vi "Script Error.vi"(0 "Error?":bool, 1 "Reset Log":bool, 2 "Error Details":string, 3 "Error Code":i32, 4 "Line Number":i32) -> ()   [LabVIEW 2013]
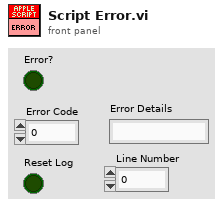
[diagram p1: front panel]
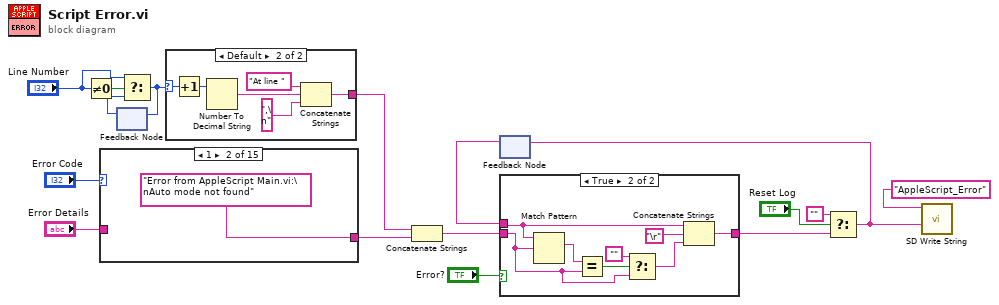
[diagram p0: block diagram]
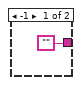
[diagram p2: hidden frame]
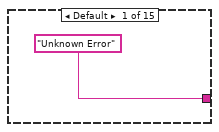
[diagram p4: hidden frame]
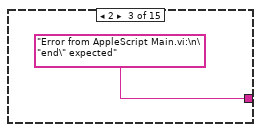
[diagram p5: hidden frame]
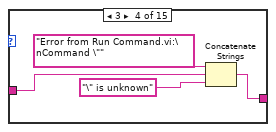
[diagram p6: hidden frame]
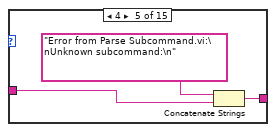
[diagram p7: hidden frame]
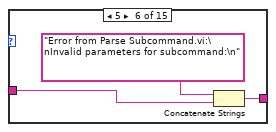
[diagram p8: hidden frame]
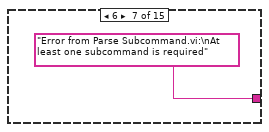
[diagram p9: hidden frame]
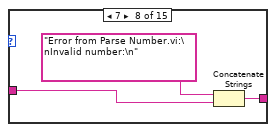
[diagram p10: hidden frame]
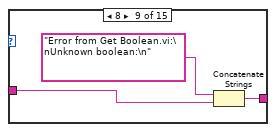
[diagram p11: hidden frame]
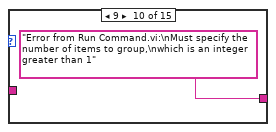
[diagram p12: hidden frame]
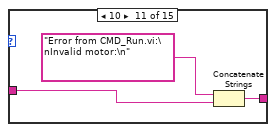
[diagram p13: hidden frame]
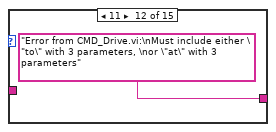
[diagram p14: hidden frame]
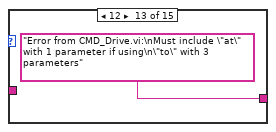
[diagram p15: hidden frame]
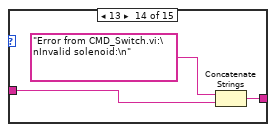
[diagram p16: hidden frame]
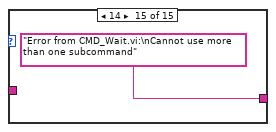
[diagram p17: hidden frame]
diagram:
  n1 = Not Equal To 0?(x="Line Number") -> (x != 0?=w4:bool)
  n2 = case shown="1" "Error Code" {
    tunnel: ["Unknown Error" "Error from AppleScript Main.vi:\nAuto mode not found" "Error from AppleScript Main.vi:\n\"end\" expected" w21 w24 w27 "Error from Parse Subcommand.vi:\nAt least one subcommand is required" w31 w34 "Error from Run Command.vi:\nMust specify the number of items to group,\nwhich is an integer greater than 1" w38 "Error from CMD_Drive.vi:\nMust include either \"to\" with 3 parameters, \nor \"at\" with 3 parameters" "Error from CMD_Drive.vi:\nMust include \"at\" with 1 parameter if using\n\"to\" with 3 parameters" w43 "Error from CMD_Wait.vi:\nCannot use more than one subcommand"] -> w9
    tunnel: "Error Details" -> [_ _ _ w22 w25 w28 _ w32 w35 _ w39 _ _ w44 _]
    frame Default {
    }
    frame 1 {
    }
    frame 2 {
    }
    frame 3 {
      n3 = Concatenate Strings("Error from Run Command.vi:\nCommand \"", w22, "\" is unknown" ("string")) -> (w21:string)
    }
    frame 4 {
      n4 = Concatenate Strings("Error from Parse Subcommand.vi:\nUnknown subcommand:\n", w25) -> (w24:string)
    }
    frame 5 {
      n5 = Concatenate Strings("Error from Parse Subcommand.vi:\nInvalid parameters for subcommand:\n", w28) -> (w27:string)
    }
    frame 6 {
    }
    frame 7 {
      n6 = Concatenate Strings("Error from Parse Number.vi:\nInvalid number:\n", w32) -> (w31:string)
    }
    frame 8 {
      n7 = Concatenate Strings("Error from Get Boolean.vi:\nUnknown boolean:\n", w35) -> (w34:string)
    }
    frame 9 {
    }
    frame 10 {
      n8 = Concatenate Strings("Error from CMD_Run.vi:\nInvalid motor:\n", w39) -> (w38:string)
    }
    frame 11 {
    }
    frame 12 {
    }
    frame 13 {
      n9 = Concatenate Strings("Error from CMD_Switch.vi:\nInvalid solenoid:\n", w44) -> (w43:string)
    }
    frame 14 {
    }
  }
  n10 = feedback #1() -> (w3:i32)  [unwired: 1 in]
  n11 = Select(t="Line Number", s=w4, f=w3) -> (s? t:f=w2:i32)
  n12 = feedback-in #1(w2) -> ()
  n13 = case shown="Default" w2 {
    selector: w2 -> [_ w49]
    tunnel: ["" w51] -> w8
    frame -1 {
    }
    frame Default {
      n14 = Increment(x=w49) -> (x+1=w48:i32)
      n15 = Number To Decimal String(number=w48) -> (decimal integer string=w53:string)  [unwired: 1 in]
      n16 = Concatenate Strings("At line " ("string"), w53, ",\n" ("string")) -> (w51:string)
    }
  }
  n17 = Concatenate Strings(w8, w9) -> (w6:string)
  n18 = feedback #2() -> (w7:string)  [unwired: 1 in]
  n19 = case shown="True" "Error?" {
    tunnel: w6 -> [_ w58]
    tunnel: w7 -> [w54 w60]
    tunnel: [w54 w62] -> w14
    frame False {
    }
    frame True {
      n20 = Match Pattern(string=w60, regular expression=w58) -> (match substring=w61:string)  [unwired: 1 in, 3 out]
      n21 = Equal?(x=w61, y=w58) -> (x = y?=w59:bool)
      n22 = Select(t="", s=w59, f=w58) -> (s? t:f=w56:string)
      n23 = Concatenate Strings(w60, "\r", w56) -> (w62:string)
    }
  }
  n24 = Select(t="", s="Reset Log", f=w14) -> (s? t:f=w13:string)
  n25 = feedback-in #2(w13) -> ()
  n26 = call <vilib>:"SD Write String.vi"("String"=w13, "Name"="AppleScript_Error") -> ()  [unwired: 8 in, 2 out]
